vi "DataAverager.vi"(6 "ImgDataArray":T1(array[cluster])) -> (2 "Averages":T2={"Centroid Avg"={"X"=239.10901, "Y"=287.93375}, "Max Intensity Avg"=0.0, "Radius Avg"={"Rx"=239.10901, "Ry"=287.93375}})   [LabVIEW 2013]
panel:
  out "Max Intensity Avg":sgl
  out "Y radius Avg":dbl
  out "X radius Avg":dbl
  out "Centroid Avg":cluster{sgl, sgl}
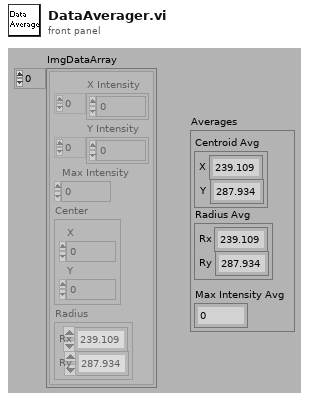
[diagram p1: front panel]
types:
  T1 = cluster{"X Intensity":u8[], "Y Intensity":u8[], "Max Intensity":sgl, "Center":cluster{"X":sgl, "Y":sgl}, "Radius":cluster{"Rx":sgl, "Ry":sgl}}[]
  T2 = cluster{"Centroid Avg":cluster{"X":sgl, "Y":sgl}, "Max Intensity Avg":sgl, "Radius Avg":cluster{"Rx":sgl, "Ry":sgl}}
  T3 = cluster{"Centroid Avg":cluster{"X":sgl, "Y":sgl}, "Max Intensity Avg":sgl, "Centroid Avg 2":cluster{"X":sgl, "Y":sgl}}
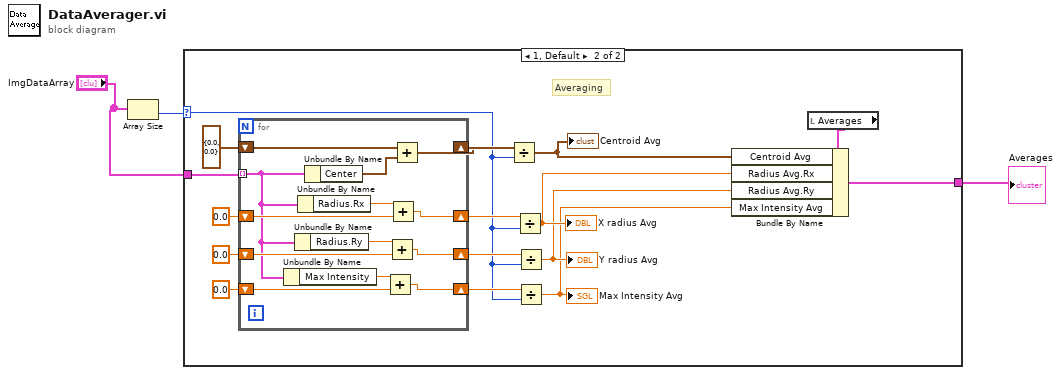
[diagram p0: block diagram]
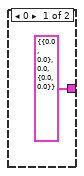
[diagram p2: hidden frame]
diagram:
  n1 = Array Size(array="ImgDataArray") -> (size(s)=w3:i32)
  n2 = case shown="1, Default" w3 {
    selector: w3 -> [_ w6]
    tunnel: "ImgDataArray" -> [_ w20]
    tunnel: [T3 {"Centroid Avg"={"X"=0.0, "Y"=0.0}, "Max Intensity Avg"=0.0, "Centroid Avg 2"={"X"=0.0, "Y"=0.0}} ("Averages") w5] -> w2
    frame 0 {
    }
    frame 1, Default {
      # "Averaging"
      n3 = for {
        tunnel: w20 -> [w21] mode=indexing
        shift-right: [w31] -> w18
        shift-left: cluster{"X Centroid":sgl, "Y Centroid":sgl} {"X Centroid"=0.0, "Y Centroid"=0.0} -> [w33]
        shift-right: [w29] -> w17
        shift-left: 0.0 -> [w28]
        shift-right: [w26] -> w14
        shift-left: 0.0 -> [w25]
        shift-right: [w23] -> w12
        shift-left: sgl 0.0 -> [w22]
        n4 = Unbundle By Name(w21) -> ("Max Intensity"=w24:sgl)
        n5 = Unbundle By Name(w21) -> ("Radius.Ry"=w27:sgl)
        n6 = Unbundle By Name(w21) -> ("Radius.Rx"=w30:sgl)
        n7 = Unbundle By Name(w21) -> ("Center"=w32:cluster{"X":sgl, "Y":sgl})
        n8 = Add(x=w24, y=w22) -> (x+y=w23:sgl)
        n9 = Add(x=w27, y=w25) -> (x+y=w26:dbl)
        n10 = Add(x=w30, y=w28) -> (x+y=w29:dbl)
        n11 = Add(x=w33, y=w32) -> (x+y=w31:cluster{sgl, sgl})
      }
      n12 = Divide(x=w18, y=w6) -> (x/y=w10:cluster{"X Centroid":sgl, "Y Centroid":sgl})
      "Centroid Avg" <- w10
      n13 = Divide(x=w17, y=w6) -> (x/y=w9:dbl)
      "X radius Avg" <- w9
      n14 = Divide(x=w14, y=w6) -> (x/y=w8:dbl)
      "Y radius Avg" <- w8
      n15 = Divide(x=w12, y=w6) -> (x/y=w7:sgl)
      "Max Intensity Avg" <- w7
      n16 = local read "Averages"() -> (w11:T2)
      n17 = Bundle By Name(cluster=w11, "Centroid Avg"=w10, "Radius Avg.Rx"=w9, "Radius Avg.Ry"=w8, "Max Intensity Avg"=w7) -> (w5:T2)
    }
  }
  "Averages" <- w2
